vi "Totalizer.vi"(9 "Period":dbl, 10 "Flow Rate":dbl, 11 "Current Total":dbl) -> (3 "New Total":dbl)   [LabVIEW 2018, in "Support Library.lvlib"]
uses:
  Support Library.lvlib
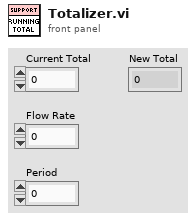
[diagram p1: front panel]
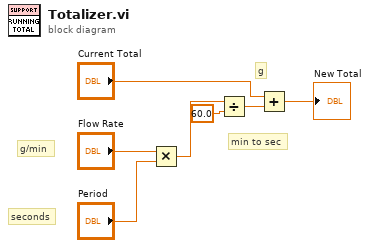
[diagram p0: block diagram]
diagram:
  # "min to sec"
  # "g"
  # "g/min"
  # "seconds"
  n1 = Multiply(x="Flow Rate", y="Period") -> (x*y=w3:dbl)
  n2 = Divide(x=w3, y=60.0) -> (x/y=w2:dbl)
  n3 = Add(x="Current Total", y=w2) -> (x+y=→"New Total":dbl)
